vi "ModuHost.vi"() -> ()   [LabVIEW 2012]
uses:
  <vilib>/userdefined/High Color/nirio_resource_hc.ctl
  hv cluster control.ctl
  <vilib>/Instr/_visa.llb/VISA Configure Serial Port (Instr).vi
  <vilib>/FPGAPlugInAG/PXI-7951R/niLvFpga_Open_PXI-7951R.vi
  <vilib>/Utility/error.llb/Error Cluster From Error Code.vi
  <vilib>/rvi/errors/niLvFpgaAdjustHostInterfaceError.vi
  <vilib>/FPGAPlugInAG/PXI-7951R/niLvFpga_Close_PXI-7951R.vi
  <vilib>/rvi/interface/nirviOpenFPGA/nirviOpenFPGA.xnode
  FPGA Bitfiles/ModuFPGAtype.ctl
  FPGA Bitfiles/ModuDAQ_FPGATarget_ModuFPGAdark_Chz-m0P+4co.lvbitx
  <vilib>/rvi/interface/nirviMethod/nirviMethod.xnode
  <vilib>/rvi/interface/nirviCloseFPGA/nirviCloseFPGA.xnode
  RT_binary.vi
  CAENHVs/CAEN/labview/CAENHVWrapper/CAENHVWrapper.lvlib
  <vilib>/FPGAPlugInAG/PXI-7951R/niLvFpga_ReadFifo_PXI-7951R.vi
  <vilib>/rvi/errors/niLvFpgaMergeErrorWithErrorCode.vi
panel:
  in  "Channel Cluster":T1={"det_type"=["", "", "", "", "", "", "", ""], "Serial numbers"=["", "", "", "", "", "", "", ""], "Sources"=["", "", "", "", "", "", "", ""], "Trigger level"=[4000, 4000, 4000, 4000, 4000, 4000, 4000, 4000], "Data Record On/Off"=[FALSE, FALSE, FALSE, FALSE, FALSE, FALSE, FALSE, FALSE, TRUE, FALSE, FALSE, FALSE, FALSE, FALSE, FALSE, TRUE], "Number of Channels"=8}
  in  "HV Cluster":T2={"HV Power On/Off"=[TRUE, TRUE], "Set Voltage"=["0", "0", "0", "0", "0", "0", "0", "0"], "HV Tolerance (%)"=1.0}
  out "created path":path
  out "File name":string
  out "Total Data Chunks to Write":dbl
  in  "Tab Control":T3(tab)
  in  "Write mode":bool
  out "directory exists - please wait":u8(slide)
  out "directory ok":bool
  in  "Write Enable":bool
  in  "File Path":path=path "D:/Users/reuterc/Desktop"
  out "File Writing Progress (%)":dbl(slide) scale=0.0..100.0
  in  "Slow Control On":bool
  in  "Fast Data On":bool
  in  "Number of Files to Write":i32=1
  in  "IP Address of NIST Time Server":string(combo)
  in  "VISA resource name":refnum<visa-resource-name>="COM3"
  in  "Rad7 Resource name":refnum<visa-resource-name>
  in  "HV Power On/Off":bool[](array[boolean])=[FALSE, FALSE, FALSE, FALSE, FALSE, FALSE, FALSE, FALSE]
  in  "HV Tolerance (%)":dbl=1.0
  out "HV":sgl[](array[numeric])
  in  "IP adress HV2":string="1_0_0"
  in  "IP adress HV1":string="0_0_0"
  in  "Set Voltage":string[](array[string])=["0", "0", "0", "0", "0", "0", "0", "0"]
  out "handle HV1":i32
  out "handle HV2":i32
  in  "General Cluster":cluster{"Location":i16} {"Location" items=["Purdue", "NIKHEF", "Zurich", "CBPF"]}
  in  "PXI address":T4 caption="RIO Device"
  in  "det_type":string[](array[combo])=["", "", "", "", "", "", "", ""]
  in  "Serial numbers":string[](array[combo])=["", "", "", "", "", "", "", ""]
  in  "Sources":string[](array[combo])=["", "", "", "", "", "", "", ""]
  in  "Trigger level":i16[](array[numeric])=[4000, 4000, 4000, 4000, 4000, 4000, 4000, 4000] caption="Trigger"
  in  "Data Record On/Off":bool[](array[boolean])=[FALSE, FALSE, FALSE, FALSE, FALSE, FALSE, FALSE, FALSE]
  in  "Testpulse Cluster":T5={"Master Pulser On/Off"=FALSE, "Testpulse Turnaround Time (samples)"=31, "Pulse Separation (samples)"=0, "Pulse duration (samples)"=0}
  out "Samples per Data Chunk":u32
  in  "DAQ Info Cluster":T6={"Data Chunks per File"=1000, "Samples per Waveform"=95, "Pretrigger Samples"=15, "circular buffer length (samples)"=1000, "Waveforms per Data Chunk"=5000} {"Waveforms per Data Chunk" format="%.2p"}
  out "Average Throughput":dbl(graph)
  out "Loop Time":u32
  out "Inst. Throughput":dbl format="%#_6p"
  out "Elements in FIFO":u32(graph)
  out "FIFO Overflow":bool
  out "Current Chunk":u32
  out "Current File":i32
  out "Data acquisition rate":dbl(graph)
  out "Waveform Graph":dynamicdata(graph)
  out "Channel number displayed":i16=-1
  in  "Arduino read rate (Hz)":dbl=1.0
  out "Slow time":u64
  out "data":dbl[](array[numeric])
  in  "XON Character":u8=17 format="%.0x"
  in  "XOFF Character":u8=19 format="%.0x"
  out "Slow Cluster":T7
  out "read buffer":string
  out "Bad sensor?":string
  in  "Max Slow Entries per File":i32=86400
  out "Current Slow File":i32
  out "Current Slow Entry":i32
  out "Slow time generated locally":bool
  out "NIST Time":u64
  out "Temperature":dbl(graph)
  out "Pressure":dbl(graph)
  out "magnetic field y coordinate":dbl(graph)
  out "total magnetic field":dbl(graph)
  out "magnetic field z coordinate":dbl(graph)
  out "magnetic field x coordinate":dbl(graph)
  out "humidity":dbl(graph)
  out "Radon":dbl(graph)
  out "XML String":string
  out "Slow XML":string
  out "error out":errorcluster
  out "UTC format":bool=TRUE
  out "Base path":path
  in  "Minutes to wait":u32=5 min=3
  out "Data Good?":bool
  out "Rad7 handle":refnum<visa-resource-name>
  out "Arduino handle":refnum<visa-resource-name>
  out "Stopped":bool
  in  "stop":bool
  # "Channel 0"
  # "Channel 1"
  # "Channel 2"
  # "Channel 3"
  # "Channel 4"
  # "Channel 5"
  # "Channel 6"
  # "Channel 7"
  # "Write continuously"
  # "Write finite number of files"
  # "Program will stop when number of Files to Write is Complete OR if stop is pressed."
  # "TODO: Make this look like the \"detectors\" tab"
  # "Waveform/Data Chunk information"
  # "To compare directly on a scope: Horizontal scale: 200 ns/div Vertical scale: ~100 mV/div If 15 pretriggers, delay = 700 ns"
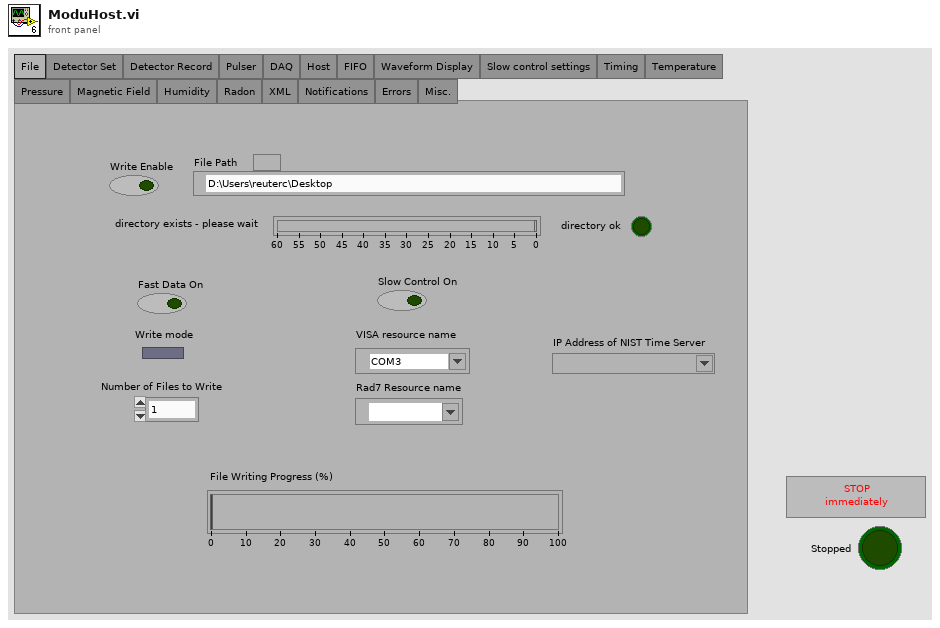
[diagram p1: front panel]
types:
  T1 = cluster{"det_type":string[], "Serial numbers":string[], "Sources":string[], "Trigger level":i16[], "Data Record On/Off":bool[], "Number of Channels":u8}
  T2 = typedef "hv cluster control.ctl" = cluster{"HV Power On/Off":bool[], "Set Voltage":string[], "HV Tolerance (%)":dbl}
  T3 = enum32{"File", "Detector Set", "Detector Record", "Pulser", "DAQ", "Host", "FIFO", "Waveform Display", "Slow control settings", "Timing", "Temperature", "Pressure", "Magnetic Field", "Humidity", "Radon", "XML", "Notifications", "Errors", "Misc."}
  T4 = typedef "nirio_resource_hc.ctl" = tag
  T5 = cluster{"Master Pulser On/Off":bool, "Testpulse Turnaround Time (samples)":u32, "Pulse Separation (samples)":u32, "Pulse duration (samples)":u32}
  T6 = cluster{"Data Chunks per File":u32, "Samples per Waveform":u32, "Pretrigger Samples":u32, "circular buffer length (samples)":u32, "Waveforms per Data Chunk":u32}
  T7 = cluster{"Arduino Parameters":dbl, "Total Number of Slow Parameters":i32, "UTC format?":bool, "Sensor Upper bounds":i32[], "Sensor Lower bounds":i32[], "Descriptions":string[], "datanames":string[]}
  T8 = enum16{"open", "replace", "create", "open or create", "replace or create", "replace or create with confirmation"}
  T9 = enum16{"Open Files", "Configure FPGA", "Data Acquisition", "Display Data", "Write Data", "Close", "Fast Off"}
  T10 = enum16{"Slow Data Off", "Initialization", "Configure", "Data Acquisition", "Data Display", "Write Data", "Close"}
  T11 = enum16{"Initialize Constants", "Open Slow Devices", "Write XML File", "Data Acqusition", "Off"}
  T12 = typedef "ModuFPGAtype.ctl" = refnum<k20>
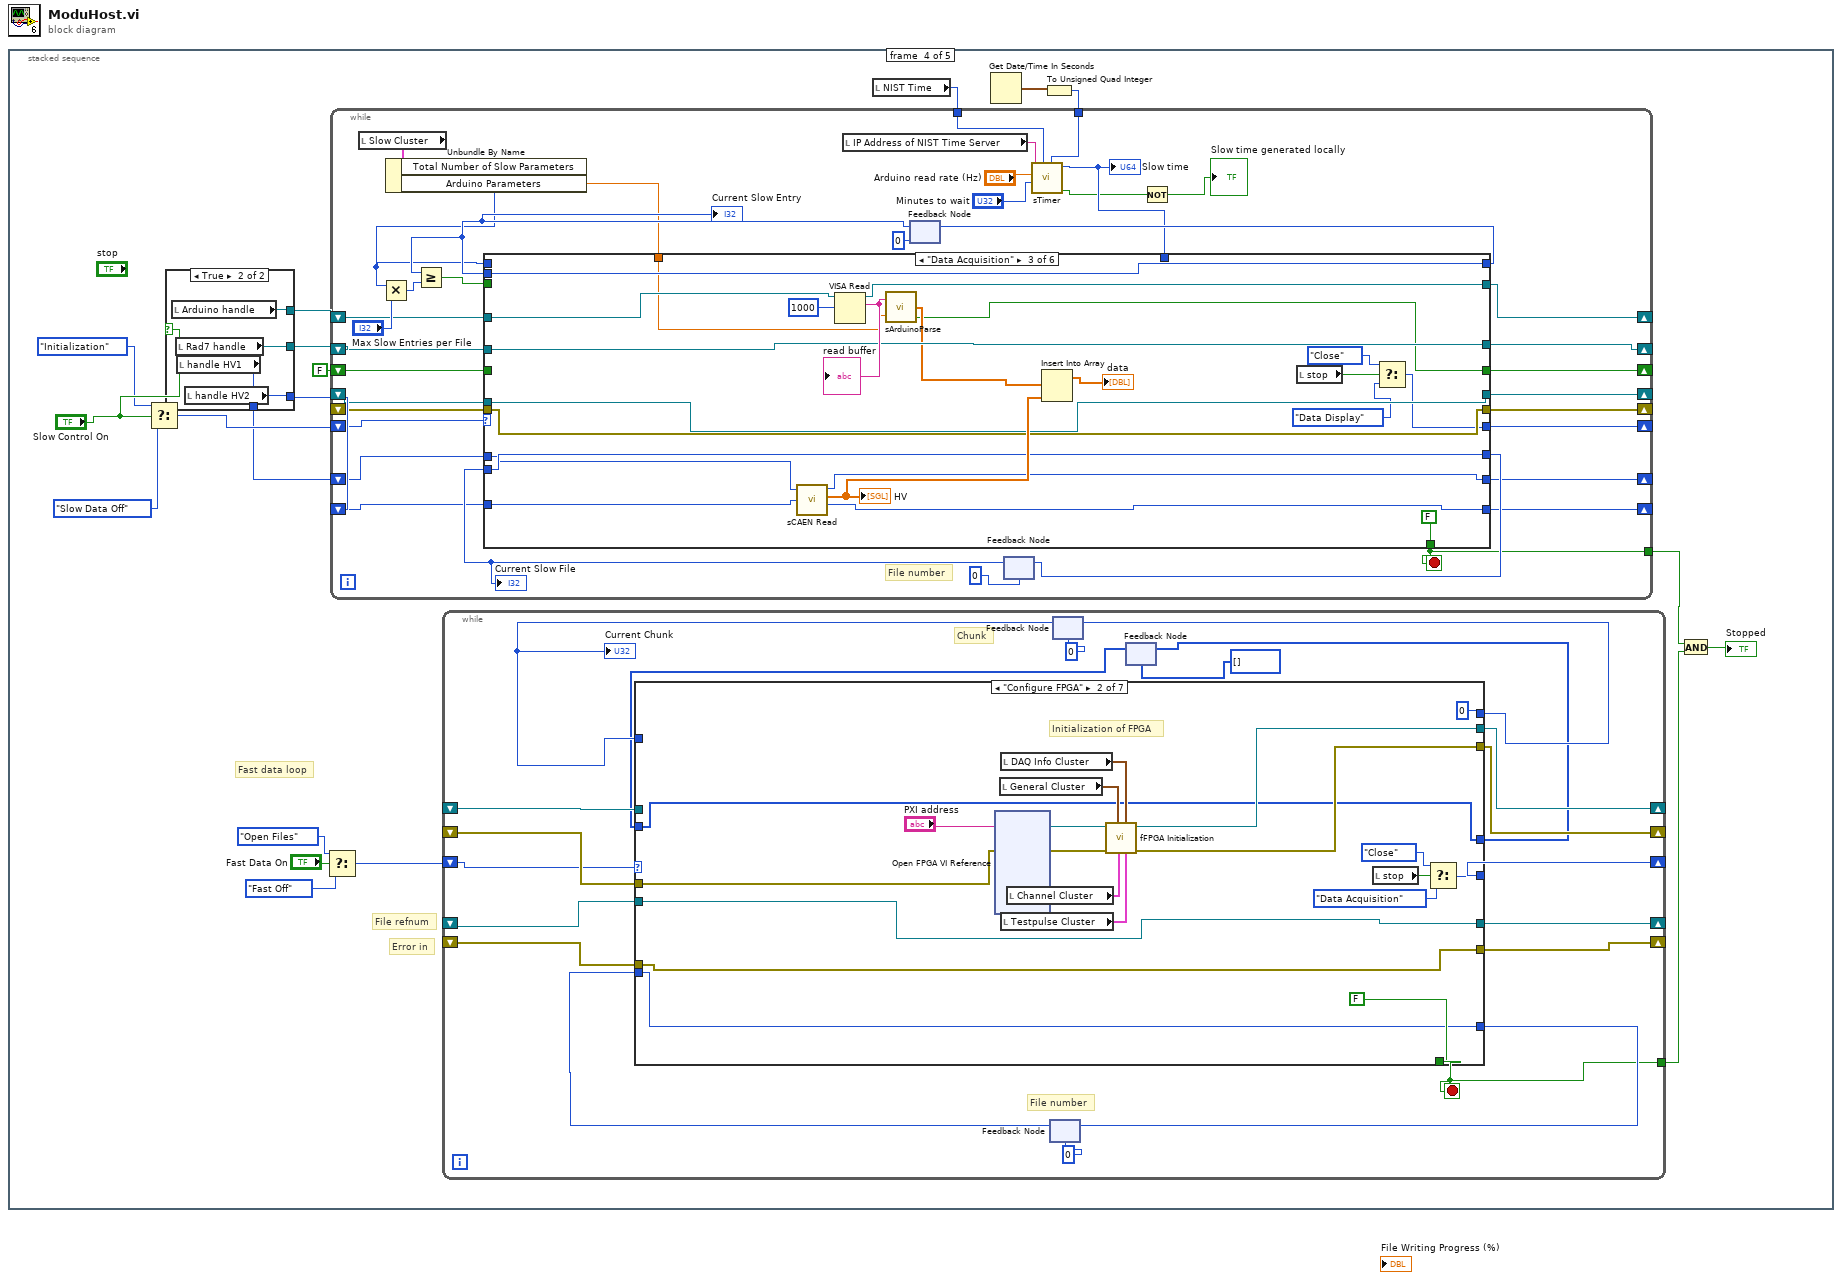
[diagram p0: block diagram]
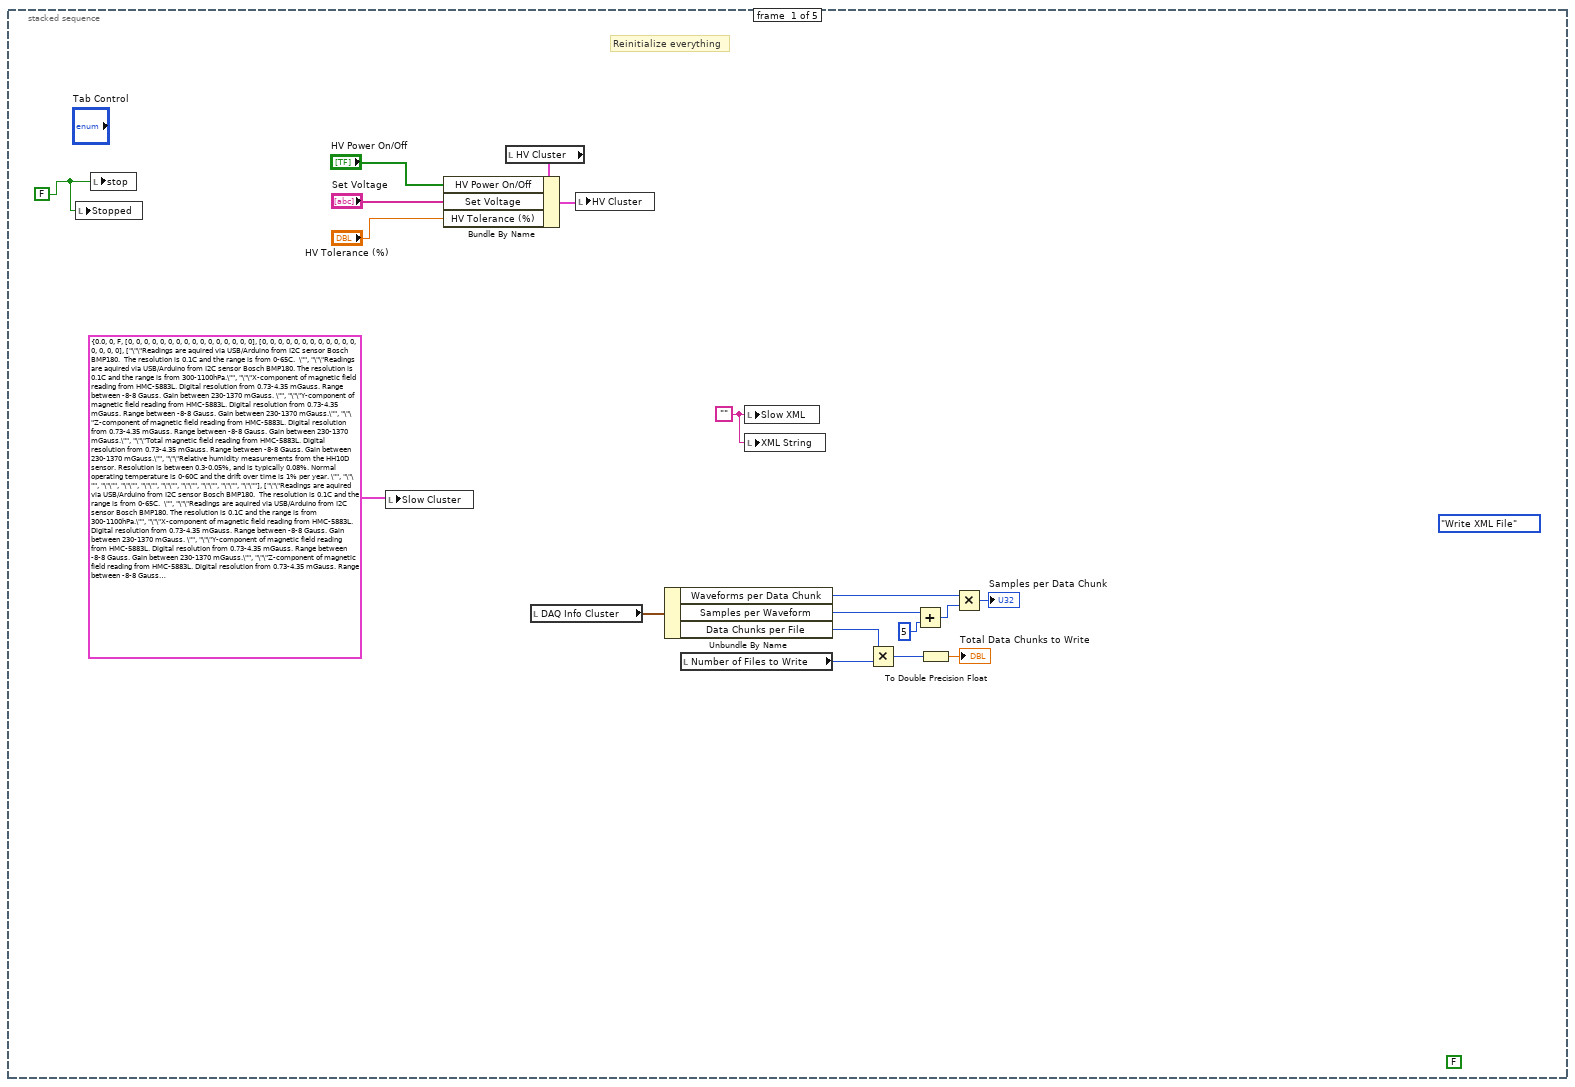
[diagram p2: hidden frame]
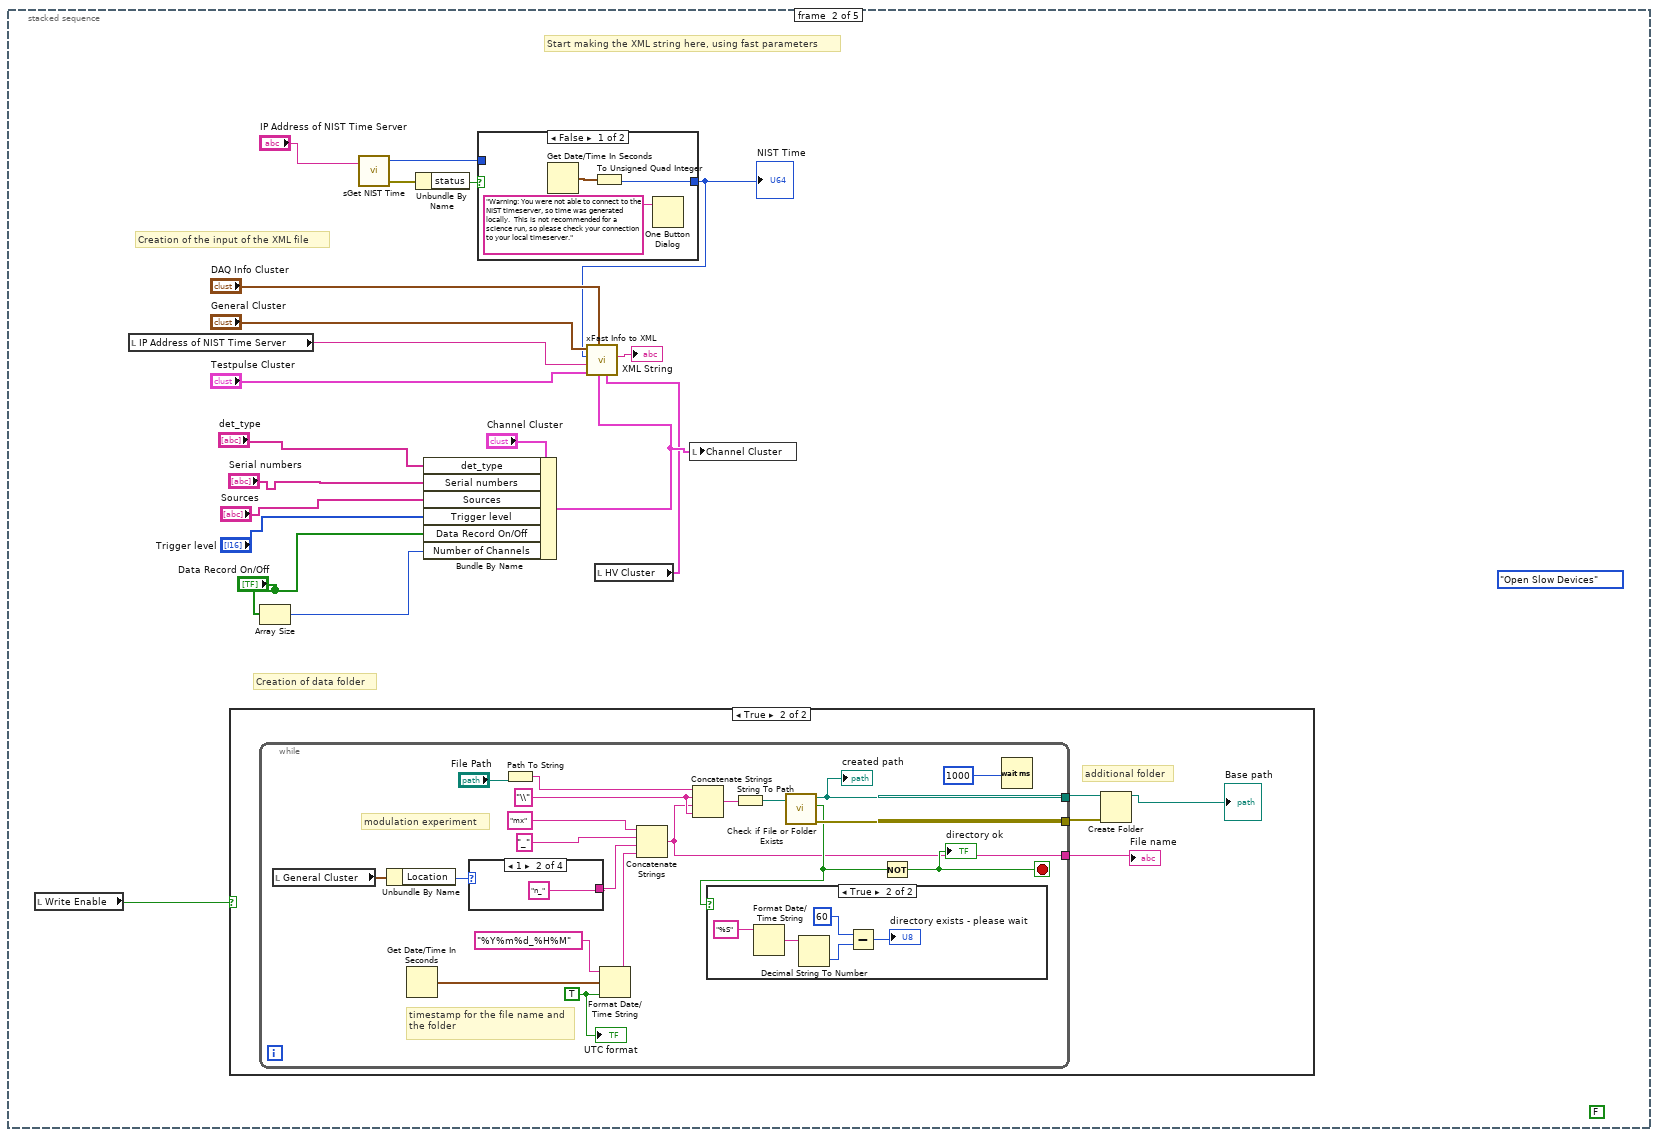
[diagram p3: hidden frame]
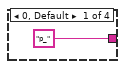
[diagram p6: hidden frame]
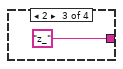
[diagram p7: hidden frame]
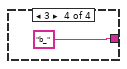
[diagram p8: hidden frame]
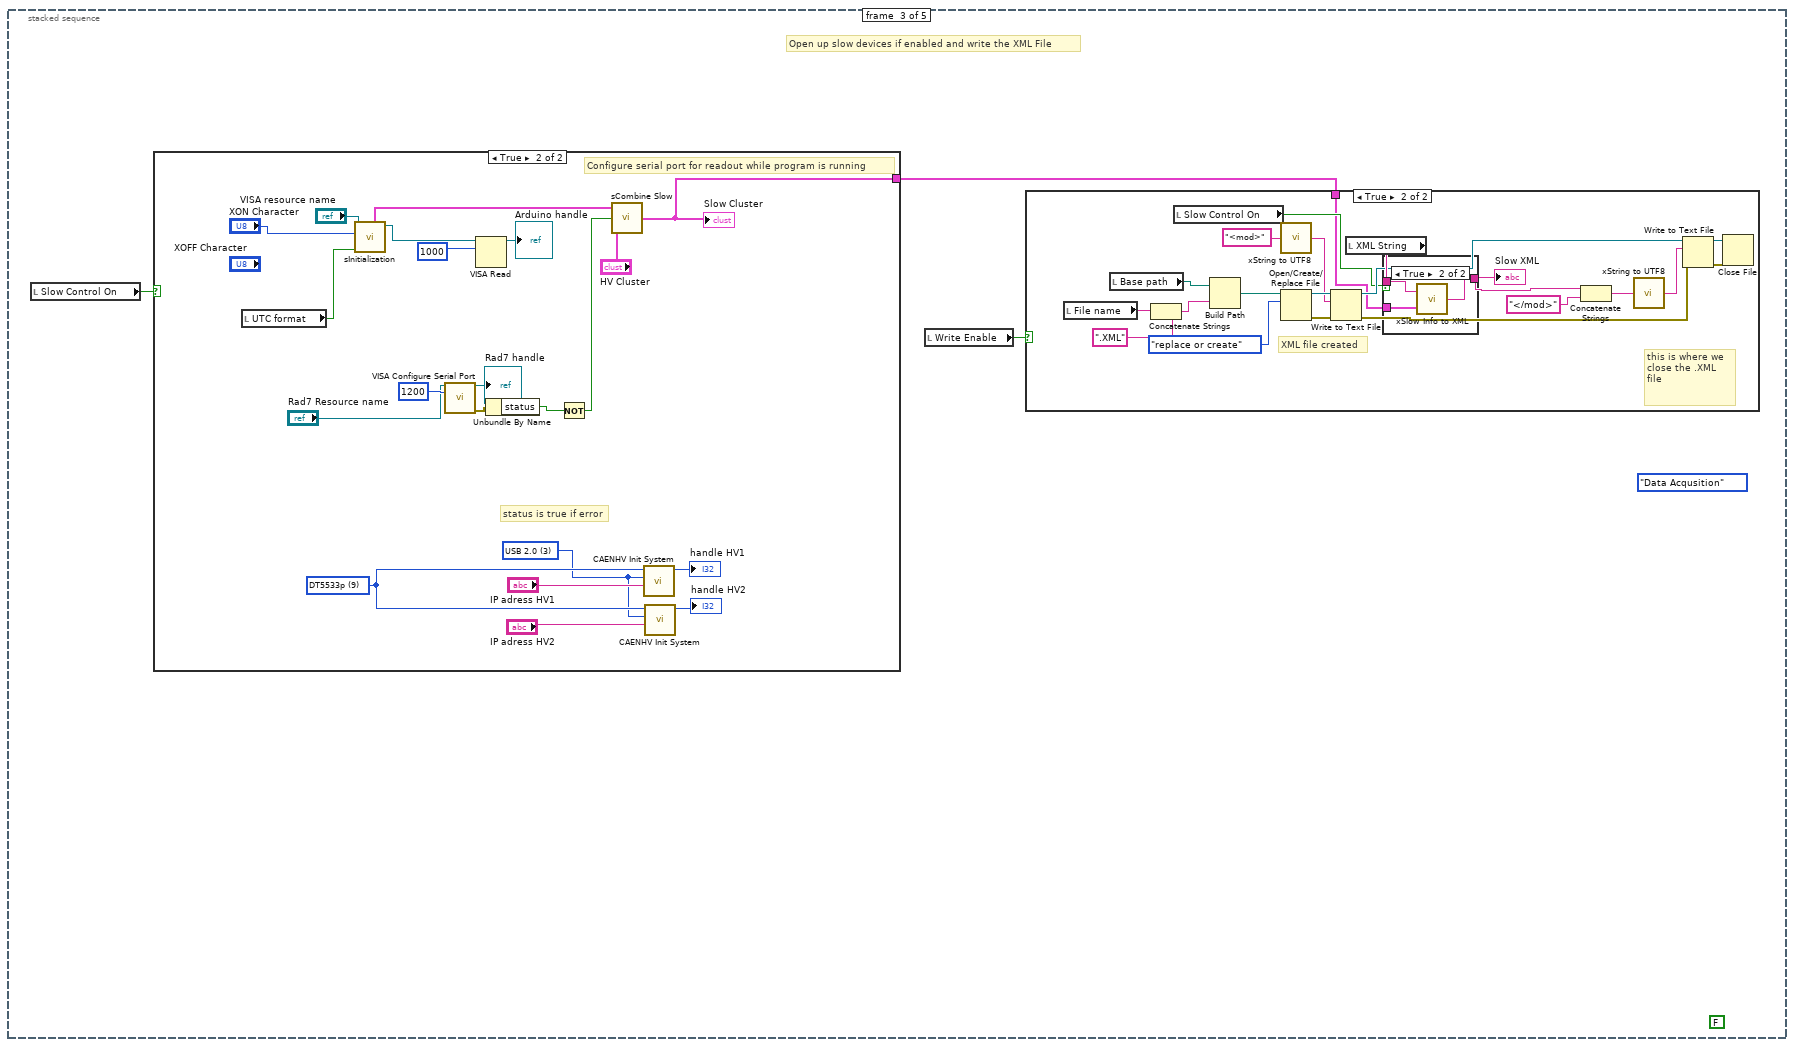
[diagram p10: hidden frame]
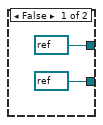
[diagram p14: hidden frame]
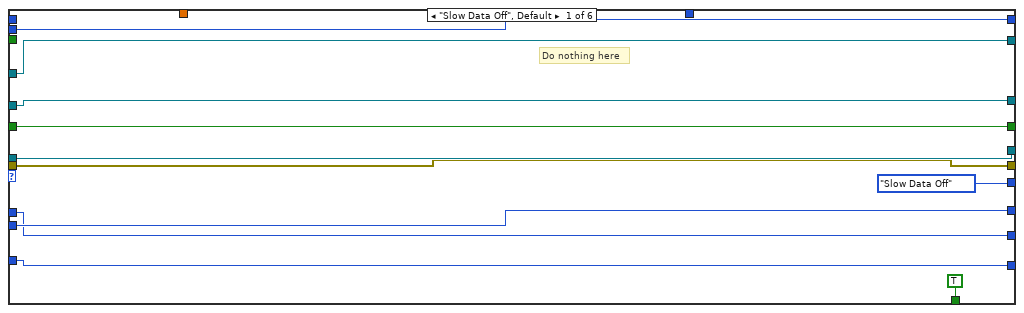
[diagram p15: hidden frame]
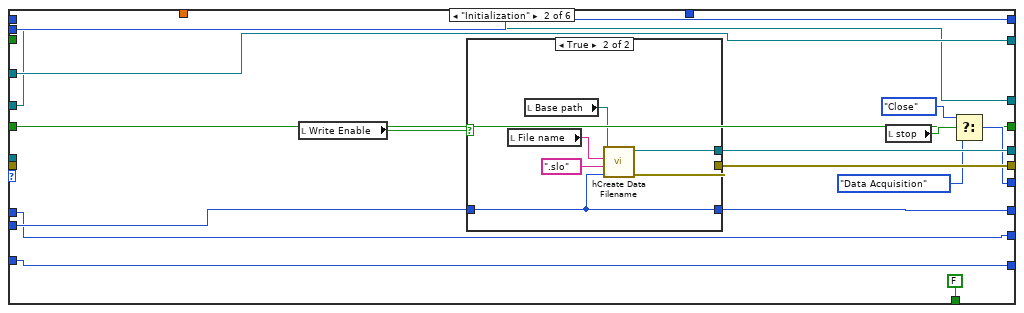
[diagram p16: hidden frame]
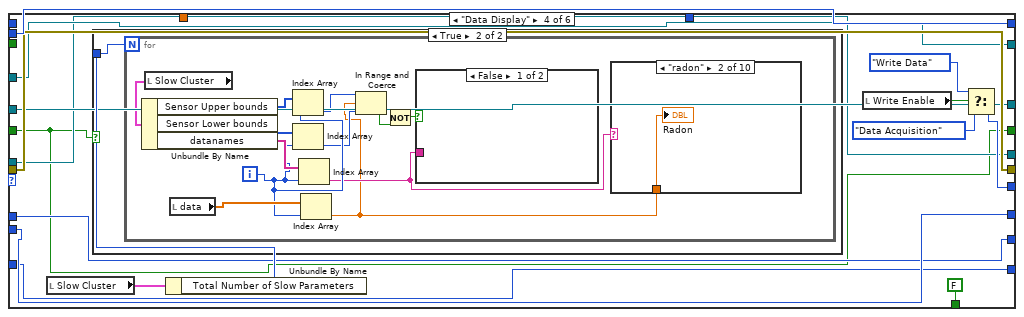
[diagram p18: hidden frame]
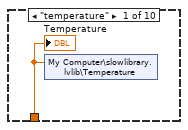
[diagram p20: hidden frame]
diagram:
  n1 = stacked-sequence {
    frame #0 {
      (unwired) FALSE
      (unwired) T11."Write XML File"
      w1 = FALSE ("stop 2")
      w17 = ""
      # "Reinitialize everything"
      n2 = local write "Stopped"(w1) -> ()
      n3 = local write "stop"(w1) -> ()
      n4 = local write "Slow Cluster"(T7 {"Arduino Parameters"=0.0, "Total Number of Slow Parameters"=0, "UTC format?"=FALSE, "Sensor Upper bounds"=[0, 0, 0, 0, 0, 0, 0, 0, 0, 0, 0, 0, 0, 0, 0, 0], "Sensor Lower bounds"=[0, 0, 0, 0, 0, 0, 0, 0, 0, 0, 0, 0, 0, 0, 0, 0], "Descriptions"=["\"\"Readings are aquired via USB/Arduino from I2C sensor Bosch BMP180.  The resolution is 0.1C and the range is from 0-65C.  \"", "\"\"Readings are aquired via USB/Arduino from I2C sensor Bosch BMP180. The resolution is 0.1C and the range is from 300-1100hPa.\"", "\"\"X-component of magnetic field reading from HMC-5883L. Digital resolution from 0.73-4.35 mGauss. Range between -8-8 Gauss. Gain between 230-1370 mGauss. \"", "\"\"Y-component of magnetic field reading from HMC-5883L. Digital resolution from 0.73-4.35 mGauss. Range between -8-8 Gauss. Gain between 230-1370 mGauss.\"", "\"\"Z-component of magnetic field reading from HMC-5883L. Digital resolution from 0.73-4.35 mGauss. Range between -8-8 Gauss. Gain between 230-1370 mGauss.\"", "\"\"Total magnetic field reading from HMC-5883L. Digital resolution from 0.73-4.35 mGauss. Range between -8-8 Gauss. Gain between 230-1370 mGauss.\"", "\"\"Relative humidity measurements from the HH10D sensor. Resolution is between 0.3-0.05%, and is typically 0.08%. Normal operating temperature is 0-60C and the drift over time is 1% per year. \"", "\"\"", "\"\"", "\"\"", "\"\"", "\"\"", "\"\"", "\"\"", "\"\"", "\"\""], "datanames"=["\"\"Readings are aquired via USB/Arduino from I2C sensor Bosch BMP180.  The resolution is 0.1C and the range is from 0-65C.  \"", "\"\"Readings are aquired via USB/Arduino from I2C sensor Bosch BMP180. The resolution is 0.1C and the range is from 300-1100hPa.\"", "\"\"X-component of magnetic field reading from HMC-5883L. Digital resolution from 0.73-4.35 mGauss. Range between -8-8 Gauss. Gain between 230-1370 mGauss. \"", "\"\"Y-component of magnetic field reading from HMC-5883L. Digital resolution from 0.73-4.35 mGauss. Range between -8-8 Gauss. Gain between 230-1370 mGauss.\"", "\"\"Z-component of magnetic field reading from HMC-5883L. Digital resolution from 0.73-4.35 mGauss. Range between -8-8 Gauss. Gain between 230-1370 mGauss.\"", "\"\"Total magnetic field reading from HMC-5883L. Digital resolution from 0.73-4.35 mGauss. Range between -8-8 Gauss. Gain between 230-1370 mGauss.\"", "\"\"Relative humidity measurements from the HH10D sensor. Resolution is between 0.3-0.05%, and is typically 0.08%. Normal operating temperature is 0-60C and the drift over time is 1% per year. \"", "\"\"", "\"\"", "\"\"", "\"\"", "\"\"", "\"\"", "\"\"", "\"\"", "\"\""]} ("Cluster")) -> ()
      n5 = local read "HV Cluster"() -> (w13:T2)
      n6 = Bundle By Name(cluster=w13, "HV Power On/Off"="HV Power On/Off", "Set Voltage"="Set Voltage", "HV Tolerance (%)"="HV Tolerance (%)") -> (w15:T2)
      n7 = local read "DAQ Info Cluster"() -> (w11:T6)
      n8 = local write "HV Cluster"(w15) -> ()
      n9 = Unbundle By Name(w11) -> ("Waveforms per Data Chunk"=w3:u32, "Samples per Waveform"=w4:u32, "Data Chunks per File"=w5:u32)
      n10 = local read "Number of Files to Write"() -> (w6:i32)
      n11 = local write "Slow XML"(w17) -> ()
      n12 = local write "XML String"(w17) -> ()
      n13 = Multiply(x=w5, y=w6) -> (x*y=w10:u32)
      n14 = Add(x=w4, y=u32 5) -> (x+y=w8:u32)
      n15 = To Double Precision Float(number=w10) -> (double precision float=→"Total Data Chunks to Write":dbl)
      n16 = Multiply(x=w3, y=w8) -> (x*y=→"Samples per Data Chunk":u32)
    }
    frame #1 {
      (unwired) FALSE
      (unwired) T11."Open Slow Devices"
      # "Start making the XML string here, using fast parameters"
      # "Creation of data folder"
      # "Creation of the input of the XML file"
      n17 = local read "Write Enable"() -> (w32:bool)
      n18 = local read "IP Address of NIST Time Server"() -> (w37:string)
      n19 = case shown="True" w32 {
        frame False {
        }
        frame True {
          # "additional folder"
          n20 = while {
            tunnel: [w59] -> w45
            tunnel: [w51] -> w46
            tunnel: [w50] -> w43
            stop <- w56 stop-if-true
            w52 = "\\" ("string")
            w62 = TRUE ("UTC format")
            # "modulation experiment"
            # "timestamp for the file name and the folder"
            n21 = local read "General Cluster"() -> (w48:cluster{"Location":i16})
            n22 = Unbundle By Name(w48) -> ("Location"=w47:i16)
            n23 = Get Date/Time In Seconds() -> (seconds since 1Jan1904=w63:timestamp)
            n24 = case shown="1" w47 {
              tunnel: ["p_" ("string") "n_" ("string") "z_" ("string") "b_"] -> w49
              frame 0, Default {
              }
              frame 1 {
              }
              frame 2 {
              }
              frame 3 {
              }
            }
            n25 = Path To String(path="File Path") -> (string=w65:string)
            n26 = Format Date/Time String(time format string (%c)="%Y%m%d_%H%M", seconds (now)=w63, UTC format=w62) -> (date/time string=w53:string)
            n27 = Concatenate Strings("mx" ("string"), "_" ("string"), w49, w53) -> (w50:string)
            n28 = Concatenate Strings(w65, w52, w50, w52) -> (w66:string)
            n29 = String To Path(string=w66) -> (path=w60:path)
            n30 = call <vilib>:"Check if File or Folder Exists.vi"("path"=w60) -> ("error out"=w59:errorcluster, "file or folder exists?"=w58:bool, "dup path"=w51:path)  [unwired: 8 in]
            "created path" <- w51
            n31 = case shown="True" w58 {
              frame False {
              }
              frame True {
                n32 = Format Date/Time String(time format string (%c)="%S") -> (date/time string=w74:string)  [unwired: 2 in]
                n33 = Decimal String To Number(string=w74) -> (number=w72:i32)  [unwired: 2 in, 1 out]
                n34 = Subtract(x=60, y=w72) -> (x-y=→"directory exists - please wait":i32)
              }
            }
            n35 = Not(x=w58) -> (.not. x?=w56:bool)
            "directory ok" <- w56
            n36 = Wait (ms)(milliseconds to wait=1000) -> ()  [unwired: 1 out]
            "UTC format" <- w62
          }
          "File name" <- w43
          n37 = Create Folder(path (use dialog)=w46, error in=w45) -> (created path=→"Base path":path)  [unwired: 1 in, 2 out]
        }
      }
      n38 = Array Size(array="Data Record On/Off") -> (size(s)=w31:i32)
      n39 = call "sGet NIST Time.vi"("IP Address of NIST Server"="IP Address of NIST Time Server") -> ("NTP Time"=w20:u64, "error out"=w22:errorcluster)  [unwired: 1 in, 1 out]
      n40 = Unbundle By Name(w22) -> ("status"=w21:bool)
      n41 = Bundle By Name(cluster="Channel Cluster", "det_type"="det_type", "Serial numbers"="Serial numbers", "Sources"="Sources", "Trigger level"="Trigger level", "Data Record On/Off"="Data Record On/Off", "Number of Channels"=w31) -> (w24:T1)
      n42 = case shown="False" w21 {
        tunnel: w20 -> [_ w42]
        tunnel: [w41 w42] -> w19
        frame False {
          n43 = Get Date/Time In Seconds() -> (seconds since 1Jan1904=w40:timestamp)
          n44 = To Unsigned Quad Integer(1:w40) -> (0:w41:u64)
          n45 = One Button Dialog(message="Warning: You were not able to connect to the NIST timeserver, so time was generated locally.  This is not recommended for a science run, so please check your connection to your local timeserver.") -> ()  [unwired: 1 in, 1 out]
        }
        frame True {
        }
      }
      "NIST Time" <- w19
      n46 = local read "HV Cluster"() -> (w23:T2)
      n47 = call "xFast Info to XML.vi"("HV Cluster"=w23, "Channel Cluster"=w24, "DAQ Info Cluster"="DAQ Info Cluster", "Testpulse Cluster"="Testpulse Cluster", "IP Address of NIST Time Server"=w37, "NIST Time"=w19, "General Cluster"="General Cluster") -> ("XML String"=→"XML String":string)  [unwired: 4 in]
      n48 = local write "Channel Cluster"(w24) -> ()
    }
    frame #2 {
      (unwired) FALSE
      (unwired) T11."Data Acqusition"
      # "Open up slow devices if enabled and write the XML File"
      n49 = local read "Slow Control On"() -> (w76:bool)
      n50 = case shown="True" w76 {
        tunnel: [_ w112] -> w78
        frame False {
        }
        frame True {
          w124 = u32 9 items=["SY1527", "SY2527", "SY4527", "SY5527", "N568", "V65XX", "N1470", "V8100", "", "DT5533p"] ("system")
          w116 = 3 items=["TCP/IP"=0, "HS CAENET"=2, "USB 2.0"=3, "CONET Optical Link"=4, "USB VCP"=5] ("LinkType")
          # "Configure serial port for readout while program is running"
          # "status is true if error"
          n51 = local read "UTC format"() -> (w105:bool)
          n52 = call "sInitialization.vi"("UTC format"=w105, "XON Character"="XON Character", "VISA resource name"="VISA resource name") -> ("VISA resource name out"=w107:refnum<visa-resource-name>, "Slow Cluster"=w104:T7)  [unwired: 6 in, 1 out]
          n53 = call-poly "VISA Configure Serial Port"("VISA resource name"="Rad7 Resource name", "baud rate (9600)"=1200) -> ("VISA resource name out"=→"Rad7 handle":refnum<visa-resource-name>, "error out"=w121:errorcluster)  [unwired: 12 in]
          n54 = VISA Read(VISA resource name=w107, byte count=u32 1000) -> (VISA resource name out=→"Arduino handle":refnum<visa-resource-name>)  [unwired: 1 in, 3 out]
          n55 = Unbundle By Name(w121) -> ("status"=w120:bool)
          n56 = Not(x=w120) -> (.not. x?=w123:bool)
          n57 = call "sCombine Slow.vi"("HV Cluster"="HV Cluster", "Rad7 On?"=w123, "Slow Cluster"=w104) -> ("Slow Cluster 2"=w112:T7)
          "Slow Cluster" <- w112
          n58 = call "CAENHV Init System.vi"("Arg"="IP adress HV1", "LinkType"=w116, "system"=w124) -> ("handle"=→"handle HV1":i32)  [unwired: 7 in, 1 out]
          n59 = call "CAENHV Init System.vi"("Arg"="IP adress HV2", "LinkType"=w116, "system"=w124) -> ("handle"=→"handle HV2":i32)  [unwired: 7 in, 1 out]
        }
      }
      n60 = local read "Write Enable"() -> (w77:bool)
      n61 = case shown="True" w77 {
        tunnel: w78 -> [_ w79]
        frame False {
        }
        frame True {
          # "XML file created"
          # "this is where we close the .XML file"
          n62 = local read "File name"() -> (w95:string)
          n63 = local read "Base path"() -> (w94:path)
          n64 = Concatenate Strings(w95, ".XML" ("substring (\"\")")) -> (w81:string)
          n65 = local read "Slow Control On"() -> (w80:bool)
          n66 = Build Path(base path=w94, name or relative path=w81) -> (appended path=w91:path)
          n67 = call "xString to UTF8.vi"("text"="<mod>") -> ("utf-8 text out"=w88:string)
          n68 = Open/Create/Replace File(file path (use dialog)=w91, operation (0:open)=T8."replace or create") -> (refnum out=w89:refnum<file>, error out=w90:errorcluster)  [unwired: 4 in, 1 out]
          n69 = Write to Text File(file (use dialog)=w89, text=w88, error in=w90) -> (refnum out=w84:refnum<file>, error out=w83:errorcluster)  [unwired: 1 in, 1 out]
          n70 = local read "XML String"() -> (w85:string)
          n71 = case shown="True" w80 {
            tunnel: [w100 w103] -> w86
            tunnel: w85 -> [w100 w102]
            tunnel: w79 -> [_ w101]
            frame False {
            }
            frame True {
              n72 = call "xSlow Info to XML.vi"("Slow Cluster"=w101, "Input String"=w102) -> ("Output String"=w103:string)
            }
          }
          "Slow XML" <- w86
          n73 = Concatenate Strings(w86, "</mod>" ("string")) -> (w96:string)
          n74 = call "xString to UTF8.vi"("text"=w96) -> ("utf-8 text out"=w99:string)
          n75 = Write to Text File(file (use dialog)=w84, text=w99, error in=w83) -> (refnum out=w98:refnum<file>, error out=w82:errorcluster)  [unwired: 1 in, 1 out]
          n76 = Close File(refnum=w98, error in=w82) -> ()  [unwired: 2 out]
        }
      }
    }
    frame #3 {
      # "Error in"
      # "File refnum"
      # "Fast data loop"
      n77 = Select(t=T10."Initialization", s="Slow Control On", f=T10."Slow Data Off") -> (s? t:f=w142:T10)
      n78 = case shown="True" "Slow Control On" {
        tunnel: [refnum<visa-resource-name> refnum ("Arduino handle") w146] -> w129
        tunnel: [refnum<visa-resource-name> refnum ("Rad7 handle") w149] -> w141
        tunnel: [_ w148] -> w140
        tunnel: [_ w147] -> w139
        frame False {
        }
        frame True {
          n79 = local read "Arduino handle"() -> (w146:refnum<visa-resource-name>)
          n80 = local read "Rad7 handle"() -> (w149:refnum<visa-resource-name>)
          n81 = local read "handle HV1"() -> (w148:i32)
          n82 = local read "handle HV2"() -> (w147:i32)
        }
      }
      n83 = Select(t=T9."Open Files", s="Fast Data On", f=T9."Fast Off") -> (s? t:f=w130:T9)
      n84 = while {
        shift-right: [w395] -> _
        shift-left: _ -> [w391]
        shift-right: [w394] -> _
        shift-left: _ -> [w390]
        shift-right: [w393] -> _
        shift-left: _ -> [w380]
        shift-right: [w392] -> _
        shift-left: _ -> [w389]
        shift-right: [w388] -> _
        shift-left: w130 -> [w379]
        tunnel: [w381] -> w137
        stop <- w381 stop-if-true
        # "File number"
        # "Chunk"
        n85 = feedback #1(0 ("f")) -> (w385:i32)
        n86 = feedback #2(u32 0 ("f")) -> (w382:u32)
        "Current Chunk" <- w382
        n87 = feedback #3(i16[] []) -> (w377:i16[])
        n88 = case shown="\"Configure FPGA\"" w379 {
          tunnel: [w406 w427 w459 w490 w522 T9."Fast Off" T9."Fast Off"] -> w388
          tunnel: [FALSE FALSE FALSE FALSE FALSE FALSE TRUE] -> w381
          tunnel: [w403 w431 w458 w486 w519 _ w590] -> w393
          tunnel: [w402 w430 w457 w485 w507 w571 w589] -> w392
          tunnel: [w401 u32 0 w456 w484 w508 w575 w588] -> w383
          tunnel: w380 -> [w403 _ w453 w486 w519 w577 w590]
          tunnel: w389 -> [w402 w416 w452 w485 w507 w576 w589]
          tunnel: w382 -> [w401 _ w451 w484 w508 w575 w588]
          tunnel: [w400 w417 w450 w483 w511 _ w587] -> w395
          tunnel: [w399 w418 w449 w482 w509 w570 w586] -> w394
          tunnel: w391 -> [_ w417 w450 w483 w512 w572 w587]
          tunnel: w390 -> [_ w418 w449 w482 w510 w573 w586]
          tunnel: w385 -> [w398 w421 w448 w481 w513 w569 w585]
          tunnel: [w398 w421 w448 w481 w506 w569 w585] -> w384
          tunnel: w377 -> [w396 w415 _ w480 w505 w568 w584]
          tunnel: [w396 w415 w442 w479 w505 w568 w584] -> w376
          frame "Open Files" {
            # "If Write Enable is on, open files"
            n89 = case shown="True" "Write Enable" {
              tunnel: [_ w412] -> w400
              tunnel: [_ w411] -> w399
              frame False {
              }
              frame True {
                n90 = local read "Base path"() -> (w410:path)
                n91 = local read "File name"() -> (w409:string)
                n92 = call "hCreate Data Filename.vi"("Combo Box"=".bin", "File name"=w409, "base path"=w410) -> ("error out"=w411:errorcluster, "refnum out"=w412:refnum<file>)  [unwired: 7 in]
              }
            }
            n93 = local read "stop"() -> (w404:bool)
            n94 = Select(t=T9."Close", s=w404, f=T9."Configure FPGA") -> (s? t:f=w406:T9)
          }
          frame "Configure FPGA" {
            # "Initialization of FPGA"
            n95 = xnode "Open FPGA VI Reference"("error in"=w416, "resource name"="PXI address") -> ("FPGA VI Reference Out"=w419:T12, "error out"=w432:errorcluster)
            n96 = local read "General Cluster"() -> (w423:cluster{"Location":i16})
            n97 = local read "DAQ Info Cluster"() -> (w424:T6)
            n98 = local read "Testpulse Cluster"() -> (w422:T5)
            n99 = local read "Channel Cluster"() -> (w414:T1)
            n100 = call "fFPGA Initialization.vi"("Testpulse Cluster"=w422, "DAQ Info Cluster"=w424, "Channel Cluster"=w414, "General Cluster"=w423, "error in"=w432, "FPGA VI Reference In"=w419) -> ("error out"=w430:errorcluster, "FPGA VI Reference Out"=w431:T12)  [unwired: 4 in]
            n101 = local read "stop"() -> (w433:bool)
            n102 = Select(t=T9."Close", s=w433, f=T9."Data Acquisition") -> (s? t:f=w427:T9)
          }
          frame "Data Acquisition" {
            # "If read times out before Number of Elements is read, Data is empty"
            n103 = local read "DAQ Info Cluster"() -> (w462:T6)
            n104 = local read "Samples per Data Chunk"() -> (w455:u32)
            n105 = Unbundle By Name(w462) -> ("Data Chunks per File"=w467:u32)
            n106 = flat-sequence {
              tunnel: [w473] -> w437
              frame #0 {
                n107 = Tick Count (ms)() -> (millisecond timer value=w472:u32)
                n108 = feedback #4(u32 0 ("millisecond timer value")) -> (w471:u32)
                n109 = feedback-in #4(w472) -> ()
                n110 = Subtract(x=w472, y=w471) -> (x-y=w473:u32)
              }
            }
            n111 = xnode "Invoke Method"("FPGA VI Reference In"=w453, "error in"=w452, "Number of Elements"=w455, "Timeout (ms)"=0) -> ("FPGA VI Reference Out"=w458:T12, "error out"=w463:errorcluster, "Data"=w442:i16[], "Elements Remaining"=w439:u32)
            "Elements in FIFO" <- w439
            n112 = Greater Or Equal?(x=w451, y=w467) -> (x >= y?=w466:bool)
            n113 = Select(t=u32 0, s=w466, f=w451) -> (s? t:f=w464:u32)
            n114 = call "fFIFO Throughput.vi"("Elements in FIFO"=w439, "Loop Time"=w437, "Array"=w442) -> ("FIFO Overflow"=→"FIFO Overflow":bool, "Inst. Throughput"=→"Inst. Throughput":dbl, "Average Throughput"=→"Average Throughput":dbl)  [unwired: 6 in]
            n115 = feedback #5(u32 500000 ("millisecond timer value")) -> (w440:u32)
            n116 = feedback-in #5(w439) -> ()
            n117 = Unbundle By Name(w463) -> ("code"=w468:i32)
            n118 = Subtract(x=w440, y=w439) -> (x-y=w438:u32)
            n119 = case shown="0, Default" w468 {
              tunnel: [w476 errorcluster {"status"=FALSE, "code"=0, "source"=""} ("error constant")] -> w457
              tunnel: w463 -> [w476 _]
              tunnel: w464 -> [w475 w477]
              tunnel: [w474 w477] -> w456
              frame 0, Default {
                n120 = Increment(x=w475) -> (x+1=w474:u32)
              }
              frame -50400 {
                # "Timeout"
              }
            }
            n121 = Divide(x=w438, y=w437) -> (x/y=w436:dbl)
            "Data acquisition rate" <- w436
            n122 = Greater Or Equal?(x=w436, y=4500000.0) -> ()  [unwired: 1 out]
            n123 = Not Equal?(x=i16[] [], y=w442) -> (x != y?=→"Data Good?":bool)
            n124 = local read "Write Enable"() -> (w454:bool)
            n125 = Select(t=T9."Write Data", s=w454, f=T9."Display Data") -> (s? t:f=w459:T9)
            "Loop Time" <- w437
          }
          frame "Display Data" {
            n126 = local read "Data Good?"() -> (w487:bool)
            n127 = case shown="True" w487 {
              tunnel: w480 -> [w493 w494]
              tunnel: [w493 w494] -> w479
              frame False {
              }
              frame True {
                # "If Fast data isn't empty and\nno data is written to a file\nthe waveform will be plotted"
                n128 = local read "Channel Cluster"() -> (w498:T1)
                n129 = local read "General Cluster"() -> (w502:cluster{"Location":i16})
                n130 = local read "DAQ Info Cluster"() -> (w500:T6)
                n131 = Unbundle By Name(w498) -> ("Trigger level"=w497:i16[])
                n132 = Unbundle By Name(w502) -> ("Location"=w501:i16)
                n133 = Unbundle By Name(w500) -> ("Samples per Waveform"=w499:u32)
                n134 = call "fDisplay Waveform.vi"("Samples per Waveform"=w499, "Location"=w501, "Trigger level"=w497, "Waveform from DAQ"=w494) -> ("Waveform Graph"=→"Waveform Graph":dynamicdata, "Channel number displayed"=→"Channel number displayed":i16)  [unwired: 6 in]
              }
            }
            n135 = local read "stop"() -> (w488:bool)
            n136 = Select(t=T9."Close", s=w488, f=T9."Data Acquisition") -> (s? t:f=w490:T9)
          }
          frame "Write Data" {
            n137 = Not Equal?(x=w505, y=i16[] []) -> (x != y?=w503:bool)
            n138 = local read "DAQ Info Cluster"() -> (w518:T6)
            n139 = Unbundle By Name(w518) -> ("Data Chunks per File"=w515:u32)
            n140 = Greater Or Equal?(x=w508, y=w515) -> (x >= y?=w516:bool)
            n141 = case shown="True" w503 {
              tunnel: "Write mode" -> [_ w538]
              tunnel: w516 -> [_ w537]
              tunnel: [FALSE w536] -> w514
              tunnel: w513 -> [w525 w535]
              tunnel: w512 -> [w528 w534]
              tunnel: [w528 w533] -> w511
              tunnel: w510 -> [w527 w532]
              tunnel: [w527 w531] -> w509
              tunnel: [w525 w530] -> w506
              tunnel: w505 -> [_ w529]
              frame False {
              }
              frame True {
                n142 = case shown="True" w537 {
                  tunnel: [w546 w556] -> w531
                  tunnel: [w545 w557] -> w533
                  tunnel: [w543 w552] -> w530
                  tunnel: [FALSE w563] -> w536
                  tunnel: w538 -> [_ w554]
                  tunnel: w535 -> [w543 w551]
                  tunnel: w534 -> [w542 w553]
                  tunnel: w532 -> [w541 w548]
                  tunnel: w529 -> [w540 w550]
                  tunnel: [w539 w549] -> _
                  frame False {
                    n143 = local read "Samples per Data Chunk"() -> (w544:u32)
                    n144 = call "fWrite Binary.vi"("error in"=w541, "Samples per data chunk"=w544, "array"=w540, "refnum in"=w542) -> ("error out"=w546:errorcluster, "refnum out"=w545:refnum<file>, "Data good?"=w539:bool)  [unwired: 5 in]
                  }
                  frame True {
                    # "opening the new ones"
                    # "closing files"
                    n145 = Increment(x=w551) -> (x+1=w552:i32)
                    n146 = local read "File name"() -> (w562:string)
                    n147 = Close File(refnum=w553, error in=w548) -> ()  [unwired: 2 out]
                    n148 = local read "Base path"() -> (w555:path)
                    n149 = call "hCreate Data Filename.vi"("File number"=w552, "Combo Box"=".bin", "File name"=w562, "base path"=w555) -> ("error out"=w559:errorcluster, "refnum out"=w560:refnum<file>)  [unwired: 6 in]
                    n150 = local read "Samples per Data Chunk"() -> (w558:u32)
                    n151 = Equal?(x=w554, y=TRUE) -> (x = y?=w567:bool)
                    n152 = Equal?(x="Number of Files to Write", y=w551) -> (x = y?=w566:bool)
                    n153 = And(x=w566, y=w567) -> (x .and. y?=w563:bool)
                    n154 = call "fWrite Binary.vi"("error in"=w559, "Samples per data chunk"=w558, "array"=w550, "refnum in"=w560) -> ("error out"=w556:errorcluster, "refnum out"=w557:refnum<file>, "Data good?"=w549:bool)  [unwired: 5 in]
                  }
                }
              }
            }
            n155 = local write "Stopped"(w514) -> ()
            n156 = local read "stop"() -> (w520:bool)
            n157 = Select(t=T9."Close", s=w520, f=T9."Data Acquisition") -> (s? t:f=w522:T9)
            "Current File" <- w513
          }
          frame "Close" {
            n158 = local read "Write Enable"() -> (w574:bool)
            n159 = case shown="True" w574 {
              tunnel: w573 -> [w580 w582]
              tunnel: w572 -> [_ w583]
              tunnel: [w580 w581] -> w570
              frame False {
              }
              frame True {
                # "Close the .bin\nfile"
                n160 = Close File(refnum=w583, error in=w582) -> (error out=w581:errorcluster)  [unwired: 1 out]
              }
            }
            n161 = xnode "Close FPGA VI Reference"("FPGA VI Reference In"=w577, "error in"=w576) -> ("error out"=w571:errorcluster)
            "error out" <- w571
          }
          frame "Fast Off", Default {
          }
        }
        n162 = feedback-in #1(w384) -> ()
        n163 = feedback-in #2(w383) -> ()
        n164 = feedback-in #3(w376) -> ()
      }
      n165 = local read "NIST Time"() -> (w125:u64)
      n166 = Get Date/Time In Seconds() -> (seconds since 1Jan1904=w127:timestamp)
      n167 = To Unsigned Quad Integer(1:w127) -> (0:w126:u64)
      n168 = while {
        shift-right: [w186] -> _
        shift-left: _ -> [w180]
        shift-right: [w181] -> _
        shift-left: _ -> [w179]
        shift-right: [w171] -> _
        shift-left: w142 -> [w172]
        shift-right: [w163] -> _
        shift-left: w129 -> [w166]
        shift-right: [w164] -> _
        shift-left: w141 -> [w165]
        shift-right: [w168] -> _
        shift-left: w140 -> [w170]
        shift-right: [w167] -> _
        shift-left: w139 -> [w169]
        tunnel: [w162] -> w138
        shift-right: [w161] -> _
        shift-left: FALSE -> [w160]
        tunnel: w126 -> [w156]
        tunnel: w125 -> [w155]
        stop <- w162 stop-if-true
        # "File number"
        n169 = local read "Slow Cluster"() -> (w174:T7)
        n170 = Unbundle By Name(w174) -> ("Total Number of Slow Parameters"=w153:i32, "Arduino Parameters"=w154:dbl)
        n171 = Multiply(x=w153, y="Max Slow Entries per File") -> (x*y=w176:i32)
        n172 = local read "IP Address of NIST Time Server"() -> (w158:string)
        n173 = feedback #6(0 ("f")) -> (w175:i32)
        "Current Slow Entry" <- w175
        n174 = Greater Or Equal?(x=w175, y=w176) -> (x >= y?=w173:bool)
        n175 = feedback #7(0 ("f")) -> (w178:i32)
        "Current Slow File" <- w178
        n176 = call "sTimer.vi"("PC Time In"=w156, "NIST Time In"=w155, "NIST Time Sync Interval (minutes)"="Minutes to wait", "Arduino read rate (Hz)"="Arduino read rate (Hz)", "IP Address of NIST Time Server"=w158) -> ("NIST Time sync'd"=w151:bool, "Slow Time"=w152:u64)  [unwired: 4 in, 1 out]
        "Slow time" <- w152
        n177 = case shown="\"Data Acquisition\"" w172 {
          tunnel: [TRUE FALSE FALSE FALSE FALSE FALSE] -> w162
          tunnel: [w190 w200 w242 w251 w291 w358] -> w163
          tunnel: [w196 w212 w234 w246 w300 w356] -> w186
          tunnel: w178 -> [w193 w210 w237 w255 w293 w363]
          tunnel: [w193 w209 w237 w255 w294 w363] -> w184
          tunnel: w175 -> [w194 w208 w236 w256 w297 w362]
          tunnel: [w194 w208 w236 w256 w296 w362] -> w182
          tunnel: [w195 w207 w235 w254 w301 w365] -> w181
          tunnel: w180 -> [w196 _ w234 w246 w299 w368]
          tunnel: w179 -> [w195 _ w235 w254 w298 w367]
          tunnel: w173 -> [_ _ _ _ w292 _]
          tunnel: [T10."Slow Data Off" w201 w225 w247 w285 T10."Slow Data Off"] -> w171
          tunnel: w170 -> [w192 w206 w232 w253 w289 w361]
          tunnel: w169 -> [w191 w205 w231 w252 w288 w360]
          tunnel: [w192 w206 w230 w253 w289 _] -> w168
          tunnel: [w191 w205 w229 w252 w288 _] -> w167
          tunnel: w166 -> [w190 w200 w233 w251 w291 w358]
          tunnel: w165 -> [w189 w199 w224 w250 w290 w357]
          tunnel: [w189 w199 w224 w250 w290 w357] -> w164
          tunnel: [w187 w198 w222 w244 w284 w355] -> w161
          tunnel: w160 -> [w187 w198 _ w244 w284 w355]
          tunnel: w154 -> [_ _ w221 _ _ _]
          tunnel: w153 -> [_ _ _ _ w283 _]
          tunnel: w152 -> [_ _ _ _ w282 _]
          frame "Slow Data Off", Default {
            # "Do nothing here"
          }
          frame "Initialization" {
            n178 = local read "Write Enable"() -> (w213:bool)
            n179 = case shown="True" w213 {
              tunnel: [_ w219] -> w212
              tunnel: w210 -> [w214 w216]
              tunnel: [w214 w216] -> w209
              tunnel: [_ w215] -> w207
              frame False {
              }
              frame True {
                n180 = local read "File name"() -> (w217:string)
                n181 = local read "Base path"() -> (w218:path)
                n182 = call "hCreate Data Filename.vi"("File number"=w216, "Combo Box"=".slo", "File name"=w217, "base path"=w218) -> ("error out"=w215:errorcluster, "refnum out"=w219:refnum<file>)  [unwired: 6 in]
              }
            }
            n183 = local read "stop"() -> (w203:bool)
            n184 = Select(t=T10."Close", s=w203, f=T10."Data Acquisition") -> (s? t:f=w201:T10)
          }
          frame "Data Acquisition" {
            n185 = call "sCAEN Read.vi"("handle HV1"=w232, "handle HV2"=w231) -> ("handle HV1 out"=w230:i32, "HV"=w239:sgl[], "handle HV2 out"=w229:i32)  [unwired: 1 in, 1 out]
            "HV" <- w239
            n186 = VISA Read(VISA resource name=w233, byte count=u32 1000) -> (VISA resource name out=w242:refnum<visa-resource-name>, read buffer=w240:string)  [unwired: 1 in, 2 out]
            "read buffer" <- w240
            n187 = call "sArduinoParse.vi"("read buffer"=w240, "Expected Arduino Parameters"=w221) -> ("Arduino Data"=w223:dbl[], "Data good?"=w222:bool)  [unwired: 2 out]
            n188 = Insert Into Array(array=w223, new element=w239) -> (→"data":dbl[])  [unwired: 1 in]
            n189 = local read "stop"() -> (w228:bool)
            n190 = Select(t=T10."Close", s=w228, f=T10."Data Display") -> (s? t:f=w225:T10)
          }
          frame "Data Display" {
            n191 = local read "Slow Cluster"() -> (w245:T7)
            n192 = Unbundle By Name(w245) -> ("Total Number of Slow Parameters"=w258:i32)
            n193 = case shown="True" w244 {
              tunnel: w258 -> [_ w260]
              frame False {
              }
              frame True {
                n194 = for {
                  N: w260 -> [_]
                  i -> [w265]
                  n195 = local read "Slow Cluster"() -> (w271:T7)
                  n196 = Unbundle By Name(w271) -> ("Sensor Upper bounds"=w270:i32[], "Sensor Lower bounds"=w269:i32[], "datanames"=w267:string[])
                  n197 = local read "data"() -> (w266:dbl[])
                  n198 = Index Array(array=w270, index=w265) -> (element=w263:i32)
                  n199 = Index Array(array=w269, index=w265) -> (element=w262:i32)
                  n200 = Index Array(array=w267, index=w265) -> (element=w264:string)
                  n201 = Index Array(array=w266, index=w265) -> (element=w261:dbl)
                  n202 = In Range and Coerce(upper limit=w263, x=w261, lower limit=w262) -> (In Range?=w272:bool)  [unwired: 1 out]
                  n203 = Not(x=w272) -> (.not. x?=w268:bool)
                  n204 = case shown="False" w268 {
                    tunnel: w264 -> [_ w281]
                    frame False {
                    }
                    frame True {
                      "Bad sensor?" <- w281
                    }
                  }
                  n205 = case shown="\"radon\"" w264 {
                    tunnel: w261 -> [w273 w274 w275 w276 w277 w278 w279 w280 _ _]
                    frame "temperature" {
                      n206 = shared-variable "My Computer\\slowlibrary.lvlib\\Temperature"(w273) -> ()  [unwired: 1 in, 1 out]
                      "Temperature" <- w273
                    }
                    frame "radon" {
                      "Radon" <- w274
                    }
                    frame "pressure" {
                      n207 = shared-variable "My Computer\\slowlibrary.lvlib\\Pressure"(w275) -> ()  [unwired: 1 in, 1 out]
                      "Pressure" <- w275
                    }
                    frame "magneticfieldx" {
                      n208 = shared-variable "My Computer\\slowlibrary.lvlib\\B_x"(w276) -> ()  [unwired: 1 in, 1 out]
                      "magnetic field x coordinate" <- w276
                    }
                    frame "magneticfieldy" {
                      n209 = shared-variable "My Computer\\slowlibrary.lvlib\\B_y"(w277) -> ()  [unwired: 1 in, 1 out]
                      "magnetic field y coordinate" <- w277
                    }
                    frame "magneticfieldz" {
                      n210 = shared-variable "My Computer\\slowlibrary.lvlib\\B_z"(w278) -> ()  [unwired: 1 in, 1 out]
                      "magnetic field z coordinate" <- w278
                    }
                    frame "magneticfieldtotal" {
                      "total magnetic field" <- w279
                    }
                    frame "humidity" {
                      n211 = shared-variable "My Computer\\slowlibrary.lvlib\\Humidity"(w280) -> ()  [unwired: 1 in, 1 out]
                      "humidity" <- w280
                    }
                    frame "seconds" {
                    }
                    frame "", Default {
                    }
                  }
                }
              }
            }
            n212 = local read "Write Enable"() -> (w259:bool)
            n213 = Select(t=T10."Write Data", s=w259, f=T10."Data Acquisition") -> (s? t:f=w247:T10)
          }
          frame "Write Data" {
            n214 = case shown="True" w284 {
              tunnel: [w305 w317] -> w301
              tunnel: [w306 w316] -> w300
              tunnel: w299 -> [w306 w315]
              tunnel: w298 -> [w305 w314]
              tunnel: w297 -> [w303 w313]
              tunnel: [w303 w312] -> w296
              tunnel: [w304 w311] -> w294
              tunnel: w293 -> [w304 w310]
              tunnel: w292 -> [_ w309]
              tunnel: w283 -> [_ w308]
              tunnel: w282 -> [_ w307]
              frame False {
              }
              frame True {
                n215 = for {
                  N: w308 -> [_]
                  tunnel: [w328] -> w317
                  tunnel: [w327] -> w316
                  tunnel: w315 -> [w326]
                  tunnel: w314 -> [w325]
                  tunnel: w313 -> [w323]
                  tunnel: [w324] -> w312
                  tunnel: [w322] -> w311
                  tunnel: w310 -> [w321]
                  tunnel: w309 -> [w320]
                  tunnel: w307 -> [w318]
                  i -> [w319]
                  n216 = case shown="False" w320 {
                    tunnel: [w338 w351] -> w327
                    tunnel: [w339 0] -> w324
                    tunnel: [w334 w348] -> w328
                    tunnel: w326 -> [w336 w347]
                    tunnel: w325 -> [w335 w346]
                    tunnel: w323 -> [w337 _]
                    tunnel: w321 -> [w333 w345]
                    tunnel: [w333 w343] -> w322
                    tunnel: w319 -> [w331 w341]
                    tunnel: w318 -> [w329 _]
                    frame False {
                      n217 = local read "data"() -> (w332:dbl[])
                      n218 = Index Array(array=w332, index=w331) -> (element=w330:dbl)
                      n219 = Increment(x=w337) -> (x+1=w339:i32)
                      n220 = call "sData Write.vi"("Slow Timestamp"=w329, "error in"=w335, "Slow Data"=w330, "Slow ID number"=w331, "File in"=w336) -> ("error out"=w334:errorcluster, "File out"=w338:refnum<file>)  [unwired: 5 in]
                    }
                    frame True {
                      # "opening the new ones"
                      # "closing files"
                      n221 = Close File(refnum=w347, error in=w346) -> ()  [unwired: 2 out]
                      n222 = local read "data"() -> (w342:dbl[])
                      n223 = local read "File name"() -> (w354:string)
                      n224 = Index Array(array=w342, index=w341) -> (element=w340:dbl)
                      n225 = local read "Base path"() -> (w349:path)
                      n226 = Increment(x=w345) -> (x+1=w343:i32)
                      n227 = call "hCreate Data Filename.vi"("File number"=w343, "Combo Box"=".slo", "File name"=w354, "base path"=w349) -> ("error out"=w352:errorcluster, "refnum out"=w350:refnum<file>)  [unwired: 6 in]
                      n228 = call "sData Write.vi"("error in"=w352, "Slow Data"=w340, "Slow ID number"=w341, "File in"=w350) -> ("error out"=w348:errorcluster, "File out"=w351:refnum<file>)  [unwired: 6 in]
                    }
                  }
                }
              }
            }
            n229 = local read "stop"() -> (w302:bool)
            n230 = Select(t=T10."Close", s=w302, f=T10."Data Acquisition") -> (s? t:f=w285:T10)
          }
          frame "Close" {
            # "Close Rad7 visa port"
            # "Close VISA port if it hasn't closed already, display error dialog in front panel"
            n231 = local read "Write Enable"() -> (w369:bool)
            n232 = case shown="False" w369 {
              tunnel: w368 -> [w372 w373]
              tunnel: w367 -> [_ w375]
              tunnel: [_ w374] -> w366
              tunnel: [w372 w373] -> w356
              frame False {
              }
              frame True {
                n233 = Close File(refnum=w373, error in=w375) -> (error out=w374:errorcluster)  [unwired: 1 out]
              }
            }
            n234 = call "CAENHV Deinit System.vi"("handle"=w361) -> ("error out"=w371:errorcluster)  [unwired: 10 in]
            n235 = call "CAENHV Deinit System.vi"("handle"=w360) -> ("error out"=w370:errorcluster)  [unwired: 10 in]
            n236 = VISA Close(VISA resource name=w358) -> ()  [unwired: 1 in, 1 out]
            n237 = Merge Errors(w366, w371, w370) -> (w365:errorcluster)
          }
        }
        n238 = feedback-in #6(w182) -> ()
        n239 = feedback-in #7(w184) -> ()
        n240 = Not(x=w151) -> (.not. x?=→"Slow time generated locally":bool)
      }
      n241 = And(x=w138, y=w137) -> (x .and. y?=→"Stopped":bool)
    }
    frame #4 {
      (unwired) T11."Off"
      (unwired) TRUE
    }
  }
